vi "Server.vi"() -> ()   [LabVIEW 2011]
uses:
  TargetData.ctl
  CommonTargetData.ctl
panel:
  out "Rsrvtn Rst Err":errorcluster
  in  "Overlord reservation timeout (hr):":i32=48
  in  "CTD":T1
  in  "XML Path":path=path "D:/Test Management/Farmer/XML/targets.xml"
  in  "Get":bool
  in  "Set":bool
  out "UI Error":errorcluster
  in  "Refresh Button":bool
  out "Target Array":T3(array[cluster])
  out "Consumer Error":errorcluster
  out "Producer Error":errorcluster
  in  "Cluster":T4
  in  "Listen Port":u16=5310
  # "Farmer Server 1.0"
  # "All Targets\nInfo"
  # "Get/Set Target Info"
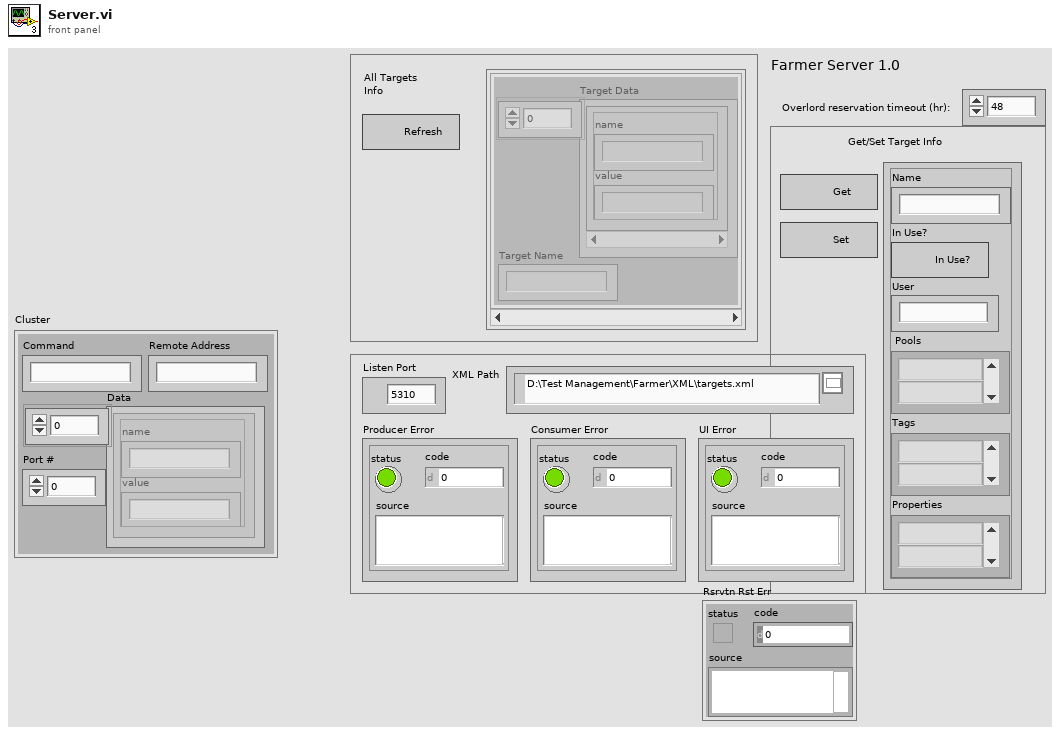
[diagram p1: front panel]
types:
  T1 = typedef "CommonTargetData.ctl" = cluster{"Name":string, "In Use?":bool, "User":string, " Pools":string[], "Tags":string[], "Properties":string[]}
  T2 = typedef "TargetData.ctl" = cluster{"name":string, "value":string}[]
  T3 = cluster{"Target Data":T2, "Target Name":string}[]
  T4 = cluster{"Data":T2, "Command":string, "Remote Address":string, "Port #":u16}
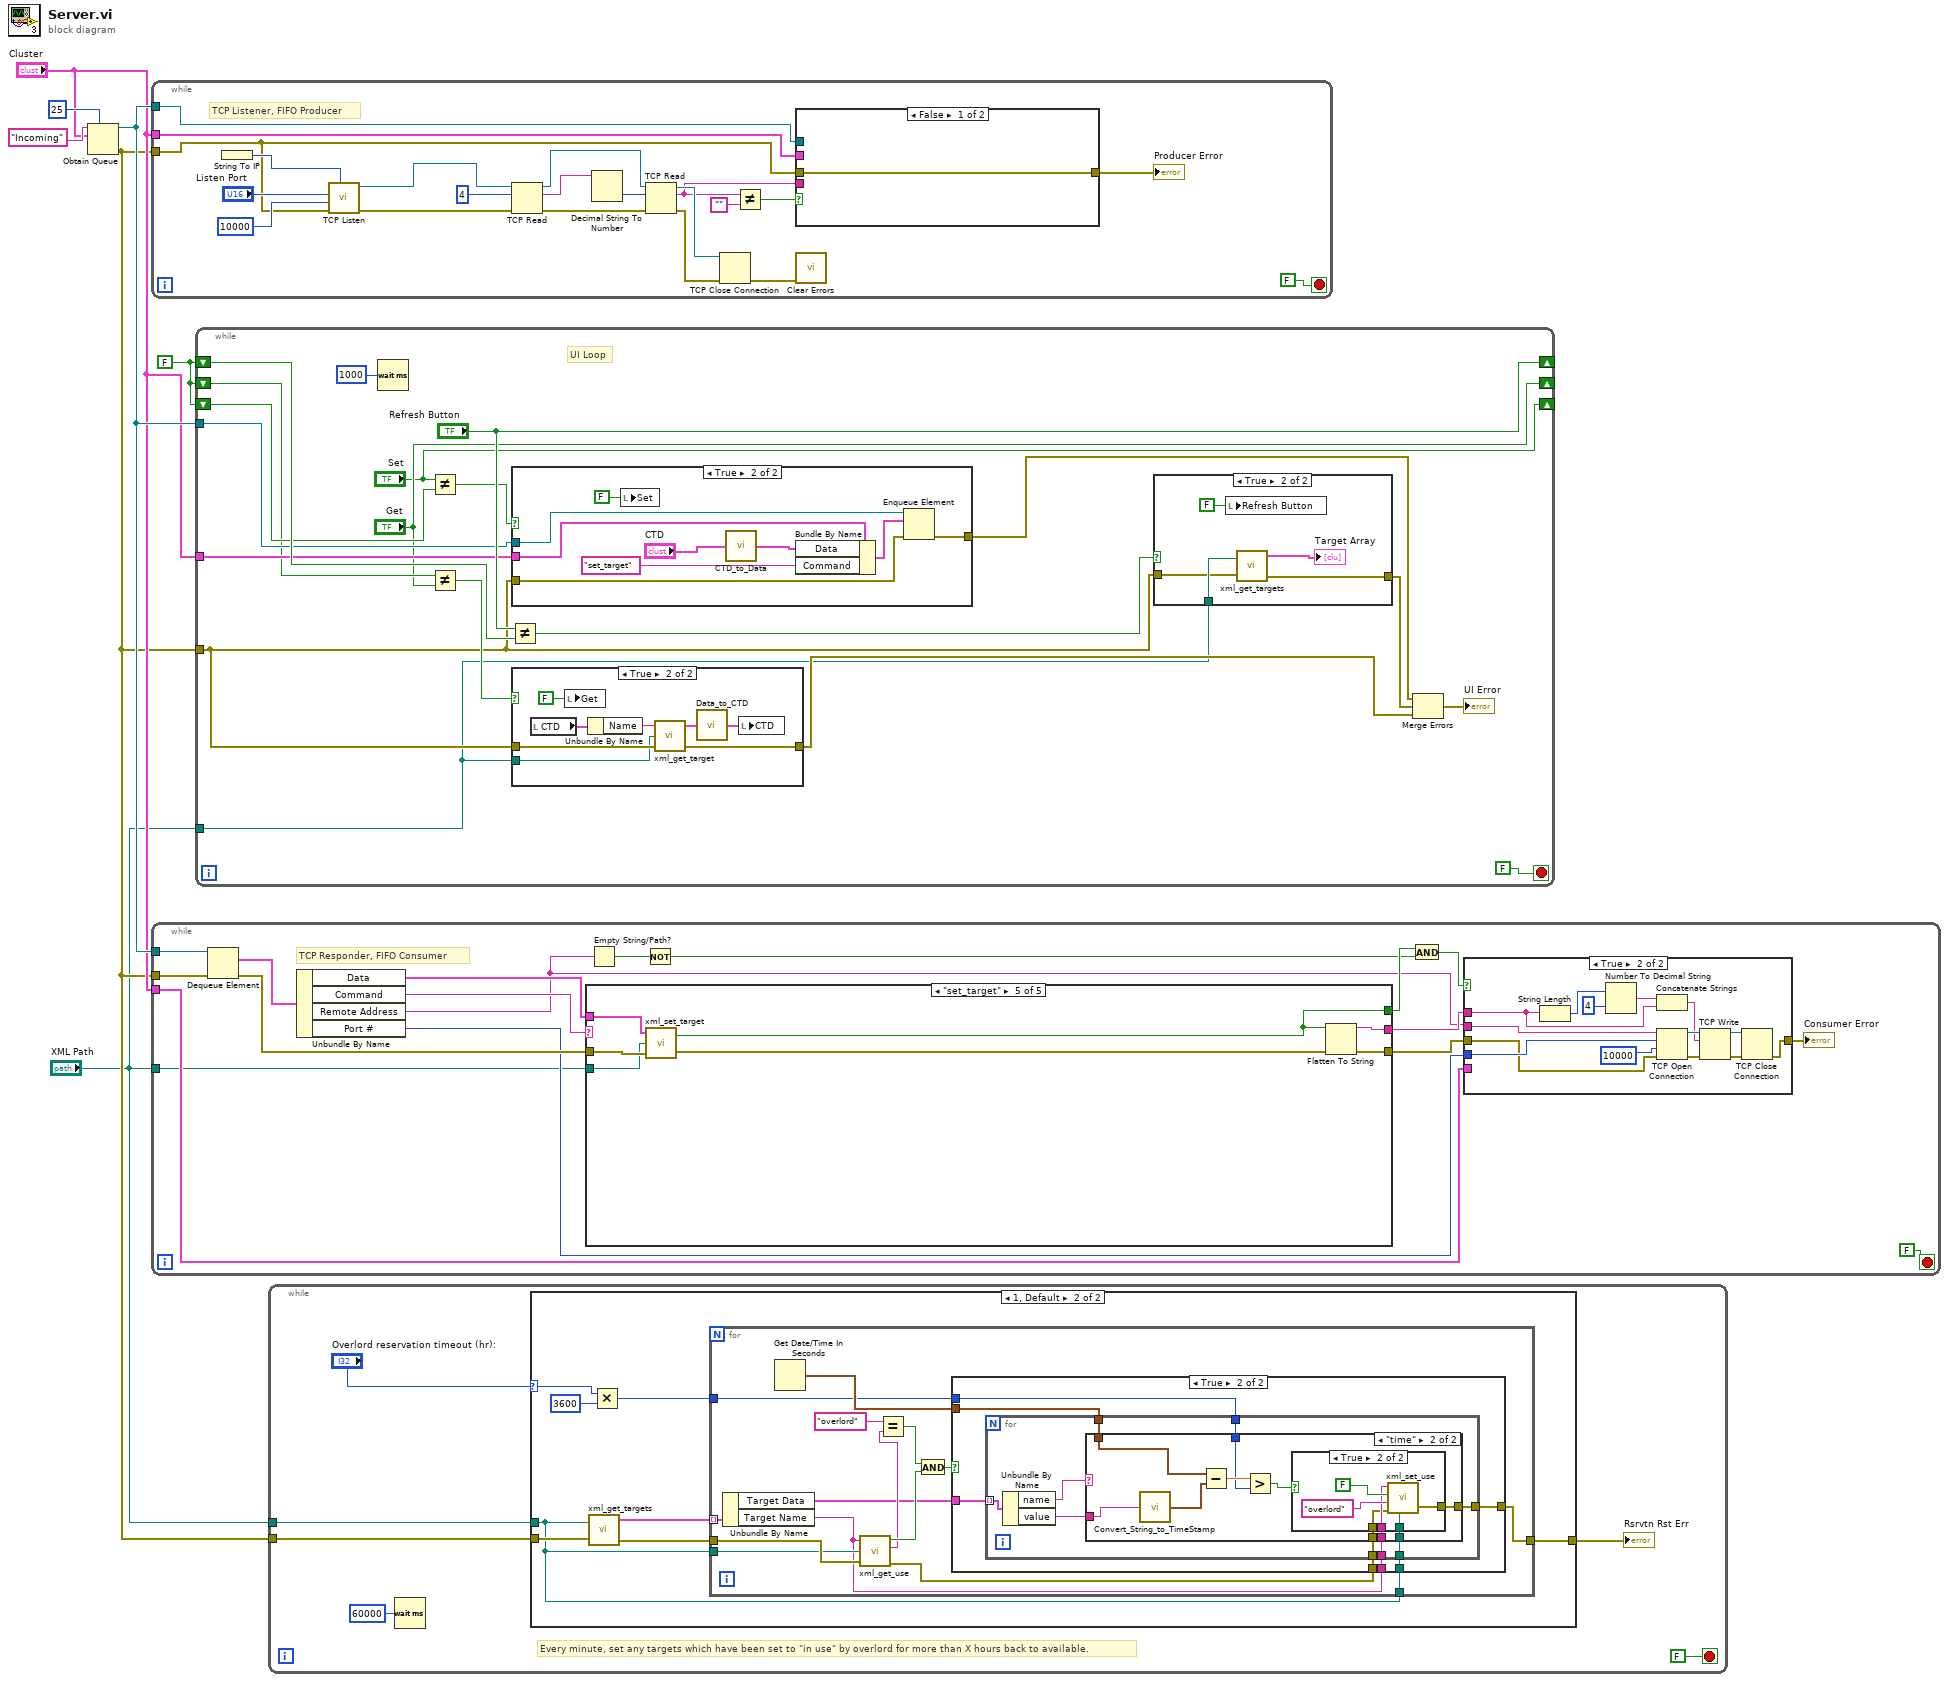
[diagram p0: block diagram]
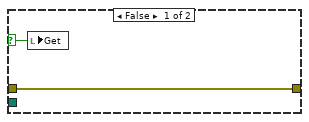
[diagram p6: hidden frame]
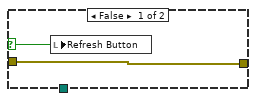
[diagram p7: hidden frame]
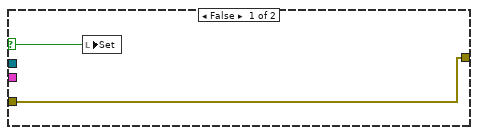
[diagram p8: hidden frame]
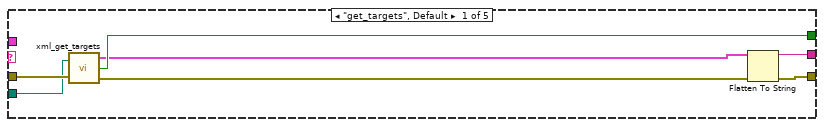
[diagram p10: hidden frame]
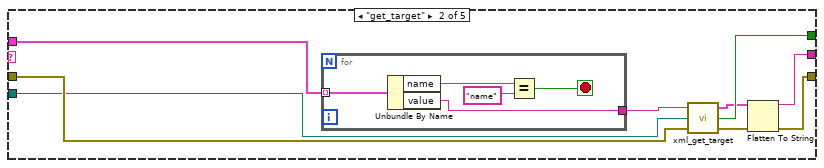
[diagram p11: hidden frame]
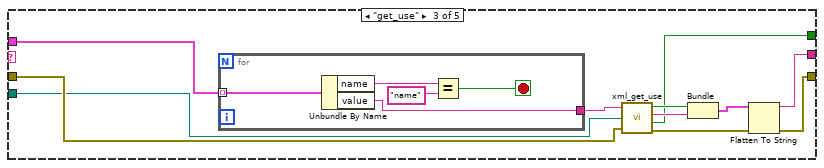
[diagram p12: hidden frame]
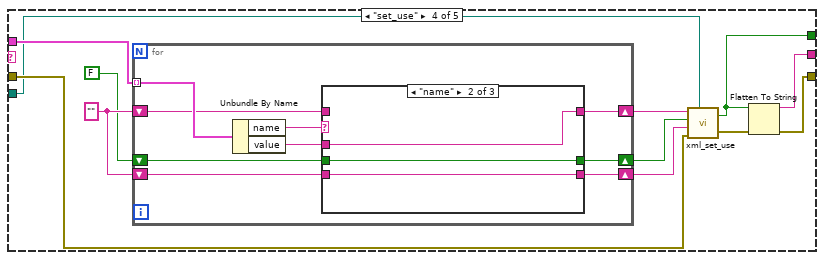
[diagram p13: hidden frame]
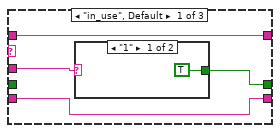
[diagram p14: hidden frame]
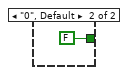
[diagram p15: hidden frame]
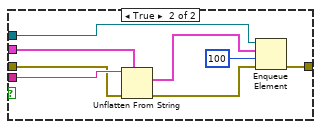
[diagram p17: hidden frame]
diagram:
  w4 = FALSE
  n1 = Obtain Queue(max queue size (-1, unlimited)=25, name (unnamed)="Incoming", element data type="Cluster") -> (queue out=w5:refnum<queue>, error out=w2:errorcluster)  [unwired: 2 in, 1 out]
  n2 = while {
    tunnel: w5 -> [w19]
    tunnel: w2 -> [w20]
    tunnel: "Cluster" -> [w18]
    stop <- FALSE stop-if-true
    # "TCP Listener, FIFO Producer"
    n3 = String To IP() -> (0:w28:u32)  [unwired: 1 in]
    n4 = call <vilib>:"TCP Listen.vi"("net address"=w28, "error in (no error)"=w20, "timeout ms (wait forever: -1)"=10000, "port"="Listen Port") -> ("error out"=w14:errorcluster, "connection ID"=w13:refnum<k5>)  [unwired: 3 in, 3 out]
    n5 = TCP Read(connection ID=w13, bytes to read=4, error in (no error)=w14) -> (connection ID out=w9:refnum<k5>, data out=w11:string, error out=w15:errorcluster)  [unwired: 1 in, 1 out]
    n6 = Decimal String To Number(string=w11) -> (number=w10:i32)  [unwired: 2 in, 1 out]
    n7 = TCP Read(connection ID=w9, bytes to read=w10, error in (no error)=w15) -> (connection ID out=w27:refnum<k5>, data out=w17:string, error out=w24:errorcluster)  [unwired: 1 in, 1 out]
    n8 = TCP Close Connection(connection ID=w27, error in (no error)=w24) -> (error out=w21:errorcluster)  [unwired: 2 out]
    n9 = Not Equal?(x=w17, y="") -> (x != y?=w22:bool)
    n10 = case shown="False" w22 {
      tunnel: w20 -> [w29 w31]
      tunnel: w19 -> [_ w37]
      tunnel: w18 -> [_ w34]
      tunnel: w17 -> [_ w33]
      tunnel: [w29 w35] -> w16
      frame False {
      }
      frame True {
        n11 = Unflatten From String(type=w34, binary string=w33, error in (no error)=w31) -> (value=w32:T4, error out=w30:errorcluster)  [unwired: 2 in, 1 out]
        n12 = Enqueue Element(queue=w37, element=w32, timeout in ms (-1)=100, error in (no error)=w30) -> (error out=w35:errorcluster)  [unwired: 2 out]
      }
    }
    "Producer Error" <- w16
    n13 = call <vilib>:"Clear Errors.vi"("error in (no error)"=w21) -> ()  [unwired: 6 in, 1 out]
  }
  n14 = while {
    tunnel: w5 -> [w55]
    tunnel: w2 -> [w54]
    tunnel: "Cluster" -> [w48]
    tunnel: "XML Path" -> [w38]
    stop <- FALSE stop-if-true
    # "TCP Responder, FIFO Consumer"
    n15 = Dequeue Element(queue=w55, error in (no error)=w54) -> (element=w53:T4, error out=w50:errorcluster)  [unwired: 1 in, 2 out]
    n16 = Unbundle By Name(w53) -> ("Data"=w51:T2, "Command"=w52:string, "Remote Address"=w41:string, "Port #"=w47:u16)
    n17 = case shown="\"set_target\"" w52 {
      tunnel: w51 -> [_ w85 w102 w119 w146]
      tunnel: w50 -> [w77 w86 w101 w118 w147]
      tunnel: [w74 w81 w95 w111 w144] -> w49
      tunnel: [w76 w83 w98 w109 w142] -> w43
      tunnel: [w73 w79 w94 w110 w143] -> w45
      tunnel: w38 -> [w71 w78 w92 w108 w141]
      frame "get_targets", Default {
        n18 = call "xml_get_targets.vi"("XML Path"=w71, "error in (no error)"=w77) -> ("Target Array"=w72:T3, "success?"=w76:bool, "error out"=w75:errorcluster)
        n19 = Flatten To String(anything=w72, error in (no error)=w75) -> (data string=w73:string, error out=w74:errorcluster)  [unwired: 2 in, 1 out]
      }
      frame "get_target" {
        n20 = for {
          tunnel: w85 -> [w91] mode=indexing
          tunnel: [w87] -> w84
          stop <- w88 stop-if-true
          n21 = Unbundle By Name(w91) -> ("name"=w90:string, "value"=w87:string)
          n22 = Equal?(x=w90, y="name") -> (x = y?=w88:bool)
        }
        n23 = call "xml_get_target.vi"("error in (no error)"=w86, "XML Path"=w78, "target name"=w84) -> ("error out"=w82:errorcluster, "success?"=w83:bool, "Data"=w80:T2)
        n24 = Flatten To String(anything=w80, error in (no error)=w82) -> (data string=w79:string, error out=w81:errorcluster)  [unwired: 2 in, 1 out]
      }
      frame "get_use" {
        n25 = for {
          tunnel: w102 -> [w107] mode=indexing
          tunnel: [w103] -> w97
          stop <- w104 stop-if-true
          n26 = Unbundle By Name(w107) -> ("name"=w106:string, "value"=w103:string)
          n27 = Equal?(x=w106, y="name") -> (x = y?=w104:bool)
        }
        n28 = call "xml_get_use.vi"("target name"=w97, "XML Path"=w92, "error in (no error)"=w101) -> ("in use?"=w100:bool, "user"=w99:string, "success?"=w98:bool, "error out"=w96:errorcluster)
        n29 = Bundle("in use?"=w100, "user"=w99) -> (w93:cluster{"in use?":bool, "user":string})  [unwired: 1 in]
        n30 = Flatten To String(anything=w93, error in (no error)=w96) -> (data string=w94:string, error out=w95:errorcluster)  [unwired: 2 in, 1 out]
      }
      frame "set_use" {
        w117 = "" ("name")
        n31 = for {
          tunnel: w119 -> [w128] mode=indexing
          shift-right: [w120] -> w113
          shift-left: w117 -> [w121]
          shift-right: [w122] -> w115
          shift-left: w117 -> [w123]
          shift-right: [w125] -> w114
          shift-left: FALSE ("success?") -> [w124]
          n32 = Unbundle By Name(w128) -> ("name"=w127:string, "value"=w126:string)
          n33 = case shown="\"name\"" w127 {
            tunnel: w126 -> [w132 w135 w138]
            tunnel: [w131 w137 w140] -> w125
            tunnel: w124 -> [_ w137 w140]
            tunnel: w123 -> [w130 _ w139]
            tunnel: [w130 w135 w139] -> w122
            tunnel: w121 -> [w129 w136 _]
            tunnel: [w129 w136 w138] -> w120
            frame "in_use", Default {
              n34 = case shown="\"1\"" w132 {
                tunnel: [TRUE ("success?") FALSE ("success?")] -> w131
                frame "1" {
                }
                frame "0", Default {
                }
              }
            }
            frame "name" {
            }
            frame "user" {
            }
          }
        }
        n35 = call "xml_set_use.vi"("target name"=w115, "in use?"=w114, "user"=w113, "error in (no error)"=w118, "XML Path"=w108) -> ("success?"=w109:bool, "error out"=w112:errorcluster)
        n36 = Flatten To String(anything=w109, error in (no error)=w112) -> (data string=w110:string, error out=w111:errorcluster)  [unwired: 2 in, 1 out]
      }
      frame "set_target" {
        n37 = call "xml_set_target.vi"("error in (no error)"=w147, "XML Path"=w141, "Data"=w146) -> ("error out"=w145:errorcluster, "success?"=w142:bool)
        n38 = Flatten To String(anything=w142, error in (no error)=w145) -> (data string=w143:string, error out=w144:errorcluster)  [unwired: 2 in, 1 out]
      }
    }
    n39 = Empty String/Path?(string/path=w41) -> (empty?=w40:bool)
    n40 = Not(x=w40) -> (.not. x?=w39:bool)
    n41 = And(x=w43, y=w39) -> (x .and. y?=w42:bool)
    n42 = case shown="True" w42 {
      tunnel: w49 -> [w56 w60]
      tunnel: w41 -> [_ w68]
      tunnel: w48 -> [_ _]
      tunnel: [w56 w65] -> w46
      tunnel: w47 -> [_ w64]
      tunnel: w45 -> [_ w59]
      frame False {
      }
      frame True {
        n43 = String Length(string=w59) -> (length=w62:i32)
        n44 = Number To Decimal String(number=w62, width (-)=i16 4) -> (decimal integer string=w58:string)
        n45 = Concatenate Strings(w58, w59) -> (w57:string)
        n46 = TCP Open Connection(address=w68, remote port or service name=w64, timeout ms (60000)=10000, error in (no error)=w60) -> (connection ID=w67:refnum<k5>, error out=w70:errorcluster)  [unwired: 1 out]
        n47 = TCP Write(connection ID=w67, data in=w57, error in (no error)=w70) -> (connection ID out=w66:refnum<k5>, error out=w69:errorcluster)  [unwired: 2 out]
        n48 = TCP Close Connection(connection ID=w66, error in (no error)=w69) -> (error out=w65:errorcluster)  [unwired: 2 out]
      }
    }
    "Consumer Error" <- w46
  }
  n49 = while {
    tunnel: w2 -> [w149]
    tunnel: w5 -> [w157]
    shift-right: ["Set"] -> _
    shift-left: w4 -> [w159]
    shift-right: ["Get"] -> _
    shift-left: w4 -> [w155]
    shift-right: ["Refresh Button"] -> _
    shift-left: w4 -> [w165]
    tunnel: "Cluster" -> [w156]
    tunnel: "XML Path" -> [w148]
    stop <- FALSE stop-if-true
    # "UI Loop"
    n50 = Wait (ms)(milliseconds to wait=u32 1000) -> ()  [unwired: 1 out]
    n51 = Not Equal?(x="Set", y=w159) -> (x != y?=w158:bool)
    n52 = Not Equal?(x=w155, y="Get") -> (x != y?=w154:bool)
    n53 = Not Equal?(x="Refresh Button", y=w165) -> (x != y?=w163:bool)
    n54 = case shown="True" w158 {
      selector: w158 -> [w184 _]
      tunnel: w149 -> [w185 w194]
      tunnel: [w185 w193] -> w161
      tunnel: w157 -> [_ w192]
      tunnel: w156 -> [_ w191]
      frame False {
        n55 = local write "Set"(w184) -> ()
      }
      frame True {
        n56 = local write "Set"(FALSE ("Set")) -> ()
        n57 = call "CTD_to_Data.vi"("CommonTargetData"="CTD") -> ("Data"=w186:T2)
        n58 = Bundle By Name(cluster=w191, "Data"=w186, "Command"="set_target") -> (w189:T4)
        n59 = Enqueue Element(queue=w192, element=w189, error in (no error)=w194) -> (error out=w193:errorcluster)  [unwired: 1 in, 2 out]
      }
    }
    n60 = case shown="True" w154 {
      selector: w154 -> [w167 _]
      tunnel: w149 -> [w168 w176]
      tunnel: [w168 w175] -> w150
      tunnel: w148 -> [_ w172]
      frame False {
        n61 = local write "Get"(w167) -> ()
      }
      frame True {
        n62 = local read "CTD"() -> (w171:T1)
        n63 = local write "Get"(FALSE ("Get")) -> ()
        n64 = Unbundle By Name(w171) -> ("Name"=w174:string)
        n65 = call "xml_get_target.vi"("error in (no error)"=w176, "XML Path"=w172, "target name"=w174) -> ("error out"=w175:errorcluster, "Data"=w170:T2)  [unwired: 1 out]
        n66 = call "Data_to_CTD.vi"("Data"=w170) -> ("CommonTargetData"=w169:T1)
        n67 = local write "CTD"(w169) -> ()
      }
    }
    n68 = case shown="True" w163 {
      selector: w163 -> [w178 _]
      tunnel: w149 -> [w177 w181]
      tunnel: [w177 w180] -> w162
      tunnel: w148 -> [_ w182]
      frame False {
        n69 = local write "Refresh Button"(w178) -> ()
      }
      frame True {
        n70 = local write "Refresh Button"(FALSE ("Refresh Button")) -> ()
        n71 = call "xml_get_targets.vi"("XML Path"=w182, "error in (no error)"=w181) -> ("Target Array"=→"Target Array":T3, "error out"=w180:errorcluster)  [unwired: 1 out]
      }
    }
    n72 = Merge Errors(w161, w162, w150) -> (→"UI Error":errorcluster)
  }
  n73 = while {
    tunnel: w2 -> [w198]
    tunnel: "XML Path" -> [w197]
    stop <- FALSE stop-if-true
    # "Every minute, set any targets which have been set to \"in use\" by overlord for more than X hours back to available."
    n74 = Wait (ms)(milliseconds to wait=u32 60000) -> ()  [unwired: 1 out]
    n75 = case shown="1, Default" "Overlord reservation timeout (hr):" {
      selector: "Overlord reservation timeout (hr):" -> [_ w206]
      tunnel: w198 -> [w201 w209]
      tunnel: w197 -> [_ w202]
      tunnel: [w201 w203] -> w196
      frame 0 {
      }
      frame 1, Default {
        n76 = call "xml_get_targets.vi"("XML Path"=w202, "error in (no error)"=w209) -> ("Target Array"=w208:T3, "error out"=w207:errorcluster)  [unwired: 1 out]
        n77 = Multiply(x=w206, y=3600) -> (x*y=w204:i32)
        n78 = for {
          tunnel: w208 -> [w224] mode=indexing
          tunnel: w207 -> [w223]
          tunnel: w202 -> [w222]
          tunnel: w204 -> [w214]
          tunnel: [w211] -> w203
          tunnel: w202 -> [w210]
          n79 = Unbundle By Name(w224) -> ("Target Data"=w216:T2, "Target Name"=w213:string)
          n80 = Get Date/Time In Seconds() -> (seconds since 1Jan1904=w215:timestamp)
          n81 = call "xml_get_use.vi"("target name"=w213, "XML Path"=w222, "error in (no error)"=w223) -> ("in use?"=w220:bool, "user"=w219:string, "error out"=w212:errorcluster)  [unwired: 1 out]
          n82 = Equal?(x="overlord", y=w219) -> (x = y?=w217:bool)
          n83 = And(x=w217, y=w220) -> (x .and. y?=w221:bool)
          n84 = case shown="True" w221 {
            tunnel: w216 -> [_ w232]
            tunnel: w215 -> [_ w231]
            tunnel: w214 -> [_ w230]
            tunnel: w213 -> [_ w229]
            tunnel: w212 -> [w225 w228]
            tunnel: [w225 w227] -> w211
            tunnel: w210 -> [_ w226]
            frame False {
            }
            frame True {
              n85 = for {
                tunnel: w232 -> [w241] mode=indexing
                tunnel: w231 -> [w238]
                tunnel: w230 -> [w237]
                tunnel: w229 -> [w236]
                tunnel: w228 -> [w235]
                tunnel: [w234] -> w227
                tunnel: w226 -> [w233]
                n86 = Unbundle By Name(w241) -> ("name"=w240:string, "value"=w239:string)
                n87 = case shown="\"time\"" w240 {
                  tunnel: w239 -> [_ w249]
                  tunnel: w238 -> [_ w252]
                  tunnel: w237 -> [_ w250]
                  tunnel: w236 -> [_ w246]
                  tunnel: w235 -> [w242 w245]
                  tunnel: [w242 w244] -> w234
                  tunnel: w233 -> [_ w243]
                  frame "other", Default {
                  }
                  frame "time" {
                    n88 = call "Convert_String_to_TimeStamp.vi"("date/time string"=w249) -> ("Resulting Time Stamp"=w248:timestamp)
                    n89 = Subtract(x=w252, y=w248) -> (x-y=w251:dbl)
                    n90 = Greater?(x=w251, y=w250) -> (0:w247:bool)
                    n91 = case shown="True" w247 {
                      tunnel: w246 -> [_ w257]
                      tunnel: w245 -> [w253 w256]
                      tunnel: [w253 w255] -> w244
                      tunnel: w243 -> [_ w254]
                      frame False {
                      }
                      frame True {
                        n92 = call "xml_set_use.vi"("target name"=w257, "in use?"=FALSE, "user"="overlord", "error in (no error)"=w256, "XML Path"=w254) -> ("error out"=w255:errorcluster)  [unwired: 1 out]
                      }
                    }
                  }
                }
              }
            }
          }
        }
      }
    }
    "Rsrvtn Rst Err" <- w196
  }
